vi "Data Channel Page.vi"(8 "error in (no error)":errorcluster, 11 "Node Ptr":T2 format="%.0x") -> (0 "error out":errorcluster)   [LabVIEW 2017, in "DSF System Explorer.lvlib"]
uses:
  DSF System Explorer.lvlib
  <vilib>/NI Veristand/Custom Device API/Custom Device Item Ref.ctl
  DSF Core.lvlibp/Classes/Component User Interface/UI Type.ctl
  <vilib>/NI Veristand/Custom Device API/Custom Device API.lvlib
  Shared/DSF Shared.lvlib
  DSF Core.lvlibp/Classes/Component User Interface/Component User Interfaces.lvclass
  DSF Core.lvlibp/Classes/User Interface/User Interface.lvclass
panel:
  in  "Tab Control":enum32{"Core", "Components"}(tab)
  in  "Default Value":dbl
  in  "Units":string
  out "Direction":enum16{"Tx", "Rx"}(ring)
  in  "Engine Data Type":T1(ring)
  in  "String Data Type":T1(ring)
  in  "String Offset":u64 format="%d bytes"
  in  "Header":cluster{"Section Name":string}={"Section Name"="Data Channel"}
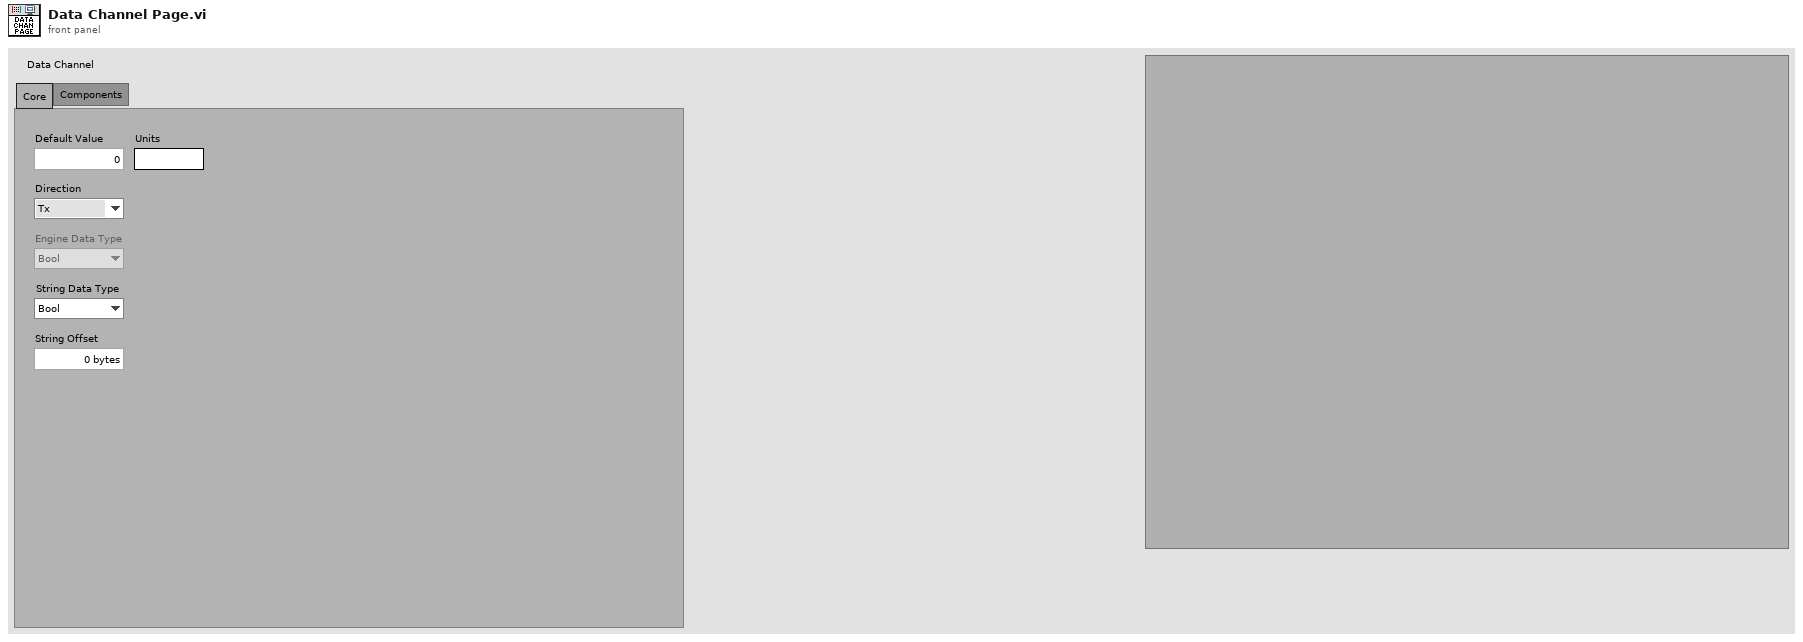
[diagram p1: front panel]
types:
  T1 = enum8{"Bool", "SGL", "DBL", "I8", "I16", "I32", "I64", "U8", "U16", "U32", "U64"}
  T2 = typedef "Custom Device API.lvlib/Custom Device Item Ref.ctl" = u64
  T3 = typedef "DSF Core.lvlibp/Component User Interfaces.lvclass/UI Type.ctl" = enum16{"Plugin", "Thread", "Rx Group", "Tx Group", "Rx Transfer", "Tx Transfer", "Rx Channel", "Tx Channel"}
  T4 = typedef "DSF Core.lvlibp/Channel Configuration.lvclass/Core Channel Configuration.ctl" = cluster{"name":string, "units":string, "engine data type":T5, "string data type":T5, "string offset":u64}
  T5 = typedef "DSF Core.lvlibp/DSF Data Type.ctl" = enum8{"Bool", "SGL", "DBL", "I8", "I16", "I32", "I64", "U8", "U16", "U32", "U64"}
  T6 = typedef "Custom Device API.lvlib/Custom Device Channel.ctl" = cluster{"Type":T7, "Units":string, "Default Value":dbl, "Faultable":bool, "Scalable":bool}
  T7 = typedef "Custom Device API.lvlib/Custom Device Channel Type.ctl" = enum16{"Input", "Output"}
  T8 = typedef "DSF Core.lvlibp/DSF Direction.ctl" = enum8{"Tx", "Rx"}
  T9 = typedef "DSF Core.lvlibp/User Interface Handler.lvclass/User Interface Ref.ctl" = refnum<vi>
  T10 = typedef "Custom Device API.lvlib/Custom Device Commands.ctl" = enum16{"Default", "Item renamed", "Shutdown", "Dynamic button pressed"}
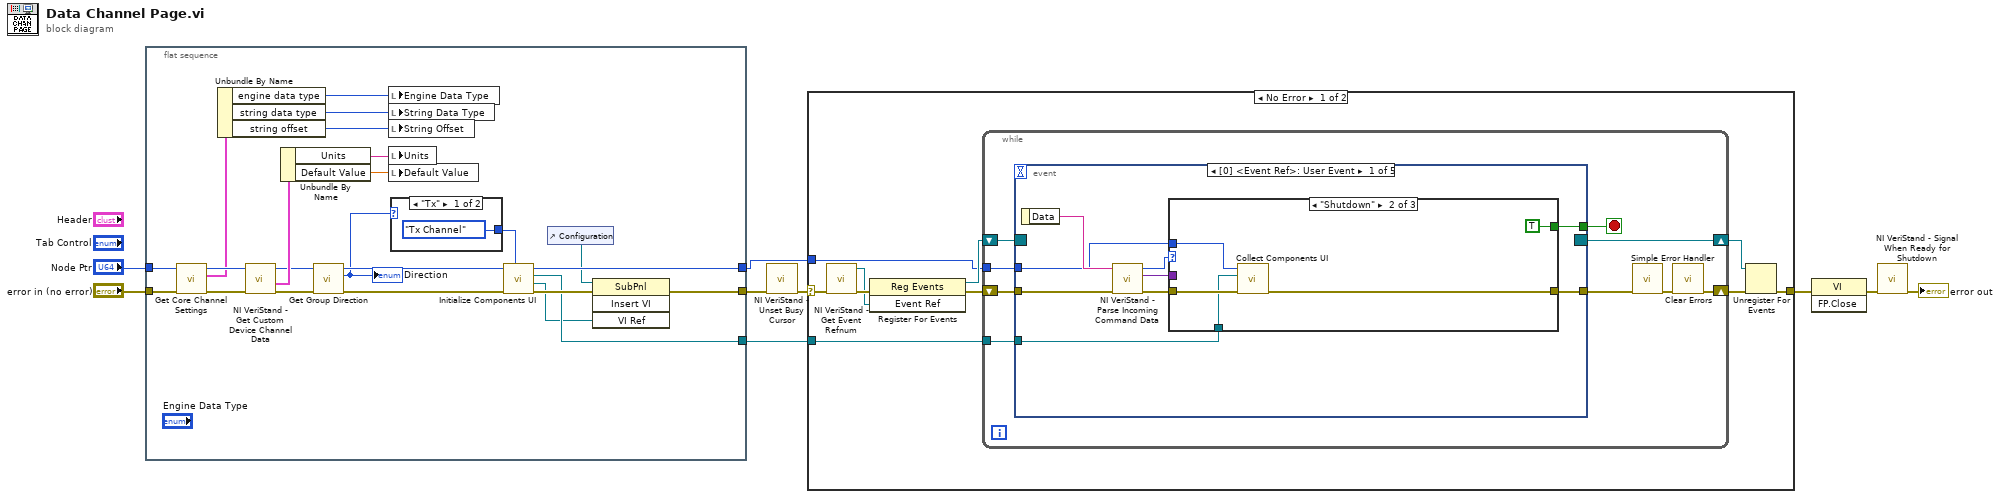
[diagram p0: block diagram]
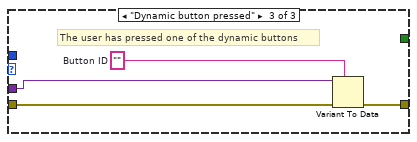
[diagram p3: hidden frame]
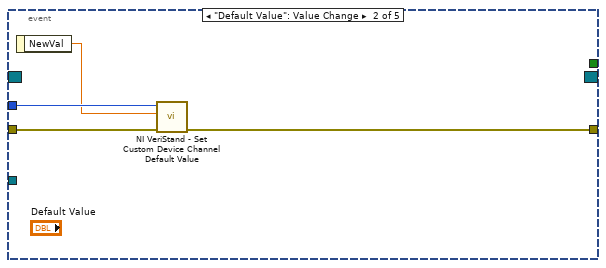
[diagram p4: hidden frame]
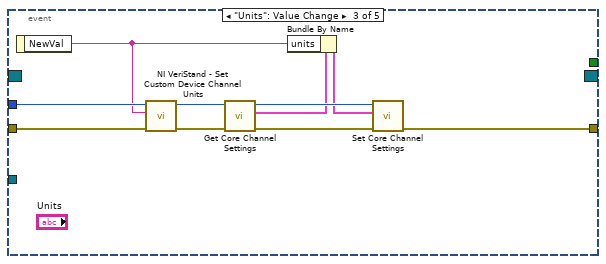
[diagram p5: hidden frame]
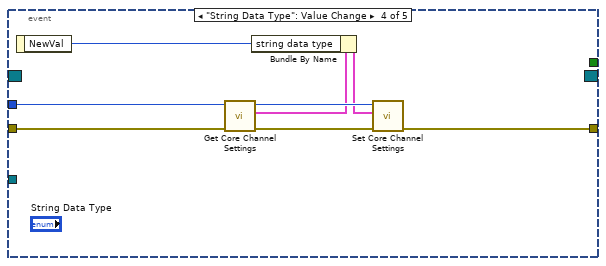
[diagram p6: hidden frame]
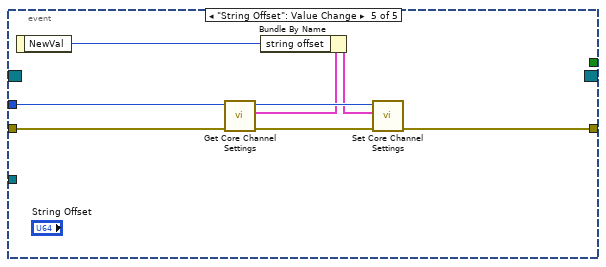
[diagram p7: hidden frame]
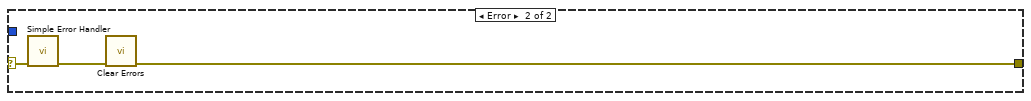
[diagram p8: hidden frame]
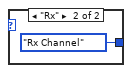
[diagram p9: hidden frame]
diagram:
  n1 = flat-sequence "Initialization code" {
    tunnel: "error in (no error)" -> [w30]
    tunnel: "Node Ptr" -> [w29]
    tunnel: [w17] -> w5
    tunnel: [w12] -> w2
    tunnel: [w13] -> w1
    frame #0 {
      n2 = call "Get Core Channel Settings.vi"("error in (no error)"=w30, "Item Ref in"=w29) -> ("error out"=w28:errorcluster, "channel configuration"=w26:T4, "Item Ref out"=w27:T2)  [unwired: 7 in]
      n3 = Unbundle By Name(w26) -> ("engine data type"=w24:T5, "string data type"=w23:T5, "string offset"=w22:u64)
      n4 = call <vilib>:"NI VeriStand - Get Custom Device Channel Data.vi"("error in (no error)"=w28, "Channel Ref in"=w27) -> ("error out"=w21:errorcluster, "Channel"=w25:T6, "Channel Ref out"=w20:T2)  [unwired: 4 in, 3 out]
      n5 = Unbundle By Name(w25) -> ("Units"=w31:string, "Default Value"=w32:dbl)
      n6 = call "Get Group Direction.vi"("error in (no error)"=w21, "Item Ref in"=w20) -> ("error out"=w16:errorcluster, "direction"=w14:T8, "Item Ref out"=w15:T2)  [unwired: 6 in, 1 out]
      "Direction" <- w14
      n7 = local write "Engine Data Type"(w24) -> ()
      n8 = local write "String Data Type"(w23) -> ()
      n9 = local write "String Offset"(w22) -> ()
      n10 = local write "Units"(w31) -> ()
      n11 = local write "Default Value"(w32) -> ()
      n12 = case shown="\"Tx\"" w14 {
        tunnel: [UI_Type."Tx Channel" ("user interface type") UI_Type."Rx Channel" ("user interface type")] -> w19
        frame "Tx" {
        }
        frame "Rx" {
        }
      }
      n13 = call "Initialize Components UI.vi"("user interface type"=w19, "error in (no error)"=w16, "Item Ref in"=w15) -> ("error out"=w18:errorcluster, "active vi"=w11:T9, "User Interface Handler"=w13:refnum<class "User Interface Handler.lvclass">, "Item Ref out"=w12:T2)  [unwired: 5 in]
      n14 = control-ref of="Configuration"() -> (w10:refnum<vi>)
      n15 = invoke class="SubPnl" method="Insert VI"(reference=w10, error in=w18, "VI Ref"=w11) -> (error out=w17:errorcluster)  [unwired: 1 in, 3 out]
    }
  }
  n16 = call <vilib>:"NI VeriStand - Unset Busy Cursor.vi"("error in (no error)"=w5) -> ("error out"=w4:errorcluster)  [unwired: 10 out]
  n17 = case shown="No Error" w4 {
    selector: w4 -> [w36 w105]
    tunnel: [w41 w103] -> w9
    tunnel: w2 -> [w37 _]
    tunnel: w1 -> [w35 _]
    frame No Error {
      n18 = call <vilib>:"NI VeriStand - Get Event Refnum.vi"("error in (no error)"=w36) -> ("error out"=w44:errorcluster, "Event Ref"=w40:refnum<user-event>)  [unwired: 9 out]
      n19 = register-events(error in=w44, w40) -> (reference out=w38:refnum<event-registration>, error out=w39:errorcluster)  [unwired: 1 in]
      n20 = while {
        tunnel: w37 -> [w49]
        shift-right: [w46] -> w42
        shift-left: w39 -> [w52]
        shift-right: [w53] -> w43
        shift-left: w38 -> [w51]
        tunnel: w35 -> [w45]
        stop <- w50 stop-if-true
        n21 = event shown="[0] <Event Ref>: User Event" {
          selector: w51 -> [_ _ _ _ _]
          dyn-events: [_ _ _ _ _] -> w53
          timeout: _ -> [_ _ _ _ _]
          tunnel: w52 -> [w62 w76 w86 w94 w102]
          tunnel: [w58 _ _ _ _] -> w50
          tunnel: [w57 w73 w77 w87 w95] -> w48
          tunnel: w49 -> [w56 w75 w85 w93 w101]
          tunnel: w45 -> [w54 _ _ _ _]
          event User Event {
            n22 = event-data() -> ("Data"=w61:string)  [unwired: 1 out]
            n23 = call <vilib>:"NI VeriStand - Parse Incoming Command Data.vi"("error in (no error)"=w62, "Incoming data"=w61) -> ("error out"=w60:errorcluster, "Outgoing data"=w55:variant, "Action"=w59:T10)  [unwired: 7 out]
            n24 = case shown="\"Shutdown\"" w59 {
              tunnel: w60 -> [w63 w67 w72]
              tunnel: [_ TRUE _] -> w58
              tunnel: [w63 w64 w69] -> w57
              tunnel: w56 -> [_ w66 _]
              tunnel: w55 -> [_ _ w71]
              tunnel: w54 -> [_ w65 _]
              frame "Default", Default {
              }
              frame "Shutdown" {
                n25 = call "Collect Components UI.vi"("error in (no error)"=w67, "User Interface Handler"=w65, "Item Ref in"=w66) -> ("error out"=w64:errorcluster)  [unwired: 7 in, 1 out]
              }
              frame "Dynamic button pressed" {
                w70 = ""  # Button ID
                # "The user has pressed one of the dynamic buttons"
                n26 = Variant To Data(error in=w72, type=w70, Variant=w71) -> (error out=w69:errorcluster)  [unwired: 1 out]
              }
            }
          }
          event "Default Value": Value Change {
            n27 = event-data() -> ("NewVal"=w74:dbl)  [unwired: 1 out]
            n28 = call <vilib>:"NI VeriStand - Set Custom Device Channel Default Value.vi"("error in (no error)"=w76, "Default Value"=w74, "Channel Ref in"=w75) -> ("error out"=w73:errorcluster)  [unwired: 7 in, 1 out]
          }
          event "Units": Value Change {
            n29 = event-data() -> ("NewVal"=w78:string)  [unwired: 1 out]
            n30 = call <vilib>:"NI VeriStand - Set Custom Device Channel Units.vi"("error in (no error)"=w86, "Units"=w78, "Channel Ref in"=w85) -> ("error out"=w84:errorcluster, "Channel Ref out"=w83:T2)  [unwired: 7 in]
            n31 = call "Get Core Channel Settings.vi"("error in (no error)"=w84, "Item Ref in"=w83) -> ("error out"=w82:errorcluster, "channel configuration"=w80:T4, "Item Ref out"=w81:T2)  [unwired: 7 in]
            n32 = Bundle By Name(cluster=w80, "units"=w78) -> (w79:T4)
            n33 = call "Set Core Channel Settings.vi"("error in (no error)"=w82, "channel configuration"=w79, "Item Ref in"=w81) -> ("error out"=w77:errorcluster)  [unwired: 7 in, 1 out]
          }
          event "String Data Type": Value Change {
            n34 = event-data() -> ("NewVal"=w88:T1)  [unwired: 1 out]
            n35 = call "Get Core Channel Settings.vi"("error in (no error)"=w94, "Item Ref in"=w93) -> ("error out"=w92:errorcluster, "channel configuration"=w90:T4, "Item Ref out"=w91:T2)  [unwired: 7 in]
            n36 = Bundle By Name(cluster=w90, "string data type"=w88) -> (w89:T4)
            n37 = call "Set Core Channel Settings.vi"("error in (no error)"=w92, "channel configuration"=w89, "Item Ref in"=w91) -> ("error out"=w87:errorcluster)  [unwired: 7 in, 1 out]
          }
          event "String Offset": Value Change {
            n38 = event-data() -> ("NewVal"=w96:u64)  [unwired: 1 out]
            n39 = call "Get Core Channel Settings.vi"("error in (no error)"=w102, "Item Ref in"=w101) -> ("error out"=w100:errorcluster, "channel configuration"=w98:T4, "Item Ref out"=w99:T2)  [unwired: 7 in]
            n40 = Bundle By Name(cluster=w98, "string offset"=w96) -> (w97:T4)
            n41 = call "Set Core Channel Settings.vi"("error in (no error)"=w100, "channel configuration"=w97, "Item Ref in"=w99) -> ("error out"=w95:errorcluster)  [unwired: 7 in, 1 out]
          }
        }
        n42 = call <vilib>:"Simple Error Handler.vi"("error in (no error)"=w48) -> ("error out"=w47:errorcluster)  [unwired: 1 in, 7 out]
        n43 = call <vilib>:"Clear Errors.vi"("error in (no error)"=w47) -> ("error out"=w46:errorcluster)  [unwired: 1 in, 5 out]
      }
      n44 = Unregister For Events(event registration refnum=w43, error in=w42) -> (error out=w41:errorcluster)
    }
    frame Error {
      n45 = call <vilib>:"Simple Error Handler.vi"("error in (no error)"=w105) -> ("error out"=w104:errorcluster)  [unwired: 1 in, 7 out]
      n46 = call <vilib>:"Clear Errors.vi"("error in (no error)"=w104) -> ("error out"=w103:errorcluster)  [unwired: 1 in, 5 out]
    }
  }
  n47 = invoke class="VI" method="FP.Close"(error in=w9) -> (error out=w8:errorcluster)  [unwired: 2 in, 2 out]
  n48 = call <vilib>:"NI VeriStand - Signal When Ready for Shutdown.vi"("error in (no error)"=w8) -> ("error out"=→"error out":errorcluster)  [unwired: 10 out]
